vi "Text2Speech.vi"(3 "TEXT TO BE SPOKEN":string="LabVIEW is the greatest software ever to be created. Next to the spork, there is no better invention!!", 4 "CHOOSE A VOICE:":i32(ring) items=["Microsoft Anna - English (United States)"], 5 "SpeechLib.ISpeechVoice":refnum<k7>) -> (1 "SpeechLib.ISpeechVoice 2":refnum<k7>)   [LabVIEW 2015]
doc: "This VI is an example of Text to Speech (TTS) using the Microsoft Speech SDK 5.1. Turn off all audio applications before running this VI.\n\n1. Enter the text to be read in the text box.\n2. Choose a voice.\n3. Run the VI.\n\nNote: The first time you run this VI, the ring control might change according to the voice order that the Speech SDK installed it in. This varies on different systems. But after the first time, the ring control remains the same.\n\nFor more information on the methods and properties, refer to the documentation that is included with the SDK or visit www.microsoft.com/speech."
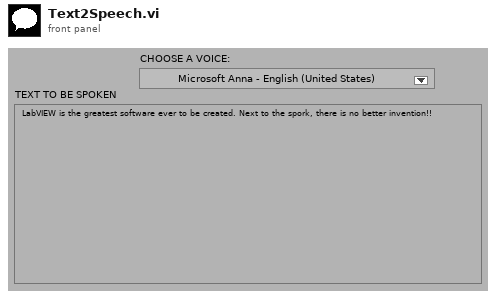
[diagram p1: front panel]
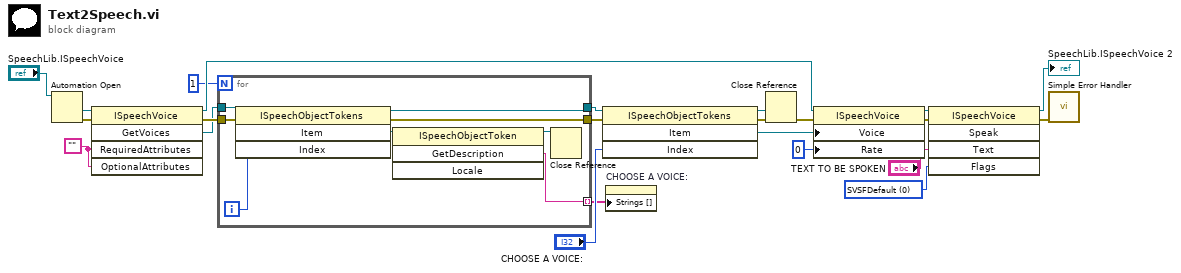
[diagram p0: block diagram]
diagram:
  w14 = ""
  w21 = 0 items=["SVSFDefault"=0, "SVSFlagsAsync"=1, "SVSFPurgeBeforeSpeak"=2, "SVSFIsFilename"=4, "SVSFIsXML"=8, "SVSFIsNotXML"=16, "SVSFPersistXML"=32, "SVSFNLPSpeakPunc, SVSFNLPMask"=64, "SVSFVoiceMask"=127, "SVSFUnusedFlags"=-128] ("Flags")
  n1 = Automation Open(Automation Refnum="SpeechLib.ISpeechVoice") -> (Automation Refnum=w22:refnum<k7>, error out=w13:errorcluster)  [unwired: 1 in, 2 out]
  n2 = invoke class="ISpeechVoice" method="GetVoices"(reference=w22, error in=w13, "RequiredAttributes"=w14, "OptionalAttributes"=w14) -> (reference out=w19:refnum<k7>, error out=w12:errorcluster, "GetVoices"=w11:refnum<k7>)  [unwired: 1 in, 2 out]
  n3 = for {
    N: 1 -> [_]
    tunnel: [w30] -> w4
    tunnel: w12 -> [w27]
    tunnel: w11 -> [w26]
    tunnel: [w25] -> w9
    tunnel: [w24] -> w8 mode=indexing
    i -> [w29]
    n4 = invoke class="ISpeechObjectTokens" method="Item"(reference=w26, error in=w27, "Index"=w29) -> (reference out=w25:refnum<k7>, error out=w30:errorcluster, "Item"=w31:refnum<k7>)  [unwired: 1 in, 1 out]
    n5 = invoke class="ISpeechObjectToken" method="GetDescription"(reference=w31) -> (reference out=w28:refnum<k7>, "GetDescription"=w24:string)  [unwired: 3 in, 2 out]
    n6 = Close Reference(reference=w28) -> ()  [unwired: 1 in, 1 out]
  }
  n7 = invoke class="ISpeechObjectTokens" method="Item"(reference=w9, error in=w4, "Index"="CHOOSE A VOICE:") -> (reference out=w5:refnum<k7>, error out=w3:errorcluster, "Item"=w15:refnum<k7>)  [unwired: 1 in, 1 out]
  n8 = property on="CHOOSE A VOICE:" class="Ring (엄격한)"("Strings []"=w8) -> ()  [unwired: 2 in, 2 out]
  n9 = Close Reference(reference=w5, error in (no error)=w3) -> (error out=w2:errorcluster)
  n10 = property class="ISpeechVoice"(reference=w19, error in=w2, "Voice"=w15, "Rate"=0) -> (reference out=w18:refnum<k7>, error out=w17:errorcluster)
  n11 = invoke class="ISpeechVoice" method="Speak"(reference=w18, error in=w17, "Text"="TEXT TO BE SPOKEN", "Flags"=w21) -> (reference out=→"SpeechLib.ISpeechVoice 2":refnum<k7>, error out=w6:errorcluster)  [unwired: 1 in, 3 out]
  n12 = call <vilib>:"Simple Error Handler.vi"("error in (no error)"=w6) -> ()  [unwired: 1 in, 8 out]
